vi "CreateIntegerArray.vi"(11 "Inputs":T1 {"Spacing" items=["Linear", "Logarithmic"]}) -> (3 "Output Array":dbl[](array[numeric]))   [LabVIEW 2014]
uses:
  <vilib>/imath/engines/lvmath2/RunTimeEngine/Managers/WorkSpace/UID Generator.vi
  <vilib>/imath/engines/lvmath2/RunTimeEngine/RunTimeType/NIMS_RunTimeType_From StrictType (excl LVString).vi
  <instcachedir>/0/NIMS_RunTimeType_From StrictType (excl LVString)_15A5391EEA9C4AACB9955AC755B83D29.lvgen/NIMS_RunTimeType_From StrictType (excl LVString)_15A5391EEA9C4AACB9955AC755B83D29_000.vi
  <vilib>/imath/engines/lvmath2/RunTimeEngine/LocalVariableDefStatement/MC_LocalVariableDefStatement_Display.vi
  <vilib>/imath/engines/lvmath2/RunTimeEngine/RangeToken/NIMS_Range.vi
  <instcachedir>/0/NIMS_Range_9BCE657718DF4976A877346C61F22738.lvgen/NIMS_Range_9BCE657718DF4976A877346C61F22738_000.vi
  <vilib>/imathl/engines/lvmath/Functions/Error Handling/Create Error.vi
  <vilib>/imath/engines/lvmath2/RunTimeEngine/Managers/SymbolTable/Clear UID.vi
  <vilib>/imath/engines/lvmath2/RunTimeEngine/NodeEndStatement/NIMS_NodeEndStatement_Output.vi
  <instcachedir>/0/NIMS_NodeEndStatement_Output_53EC0D466D134D7ABD903AC30B43404B.lvgen/NIMS_NodeEndStatement_Output_53EC0D466D134D7ABD903AC30B43404B_005.vi
  <vilib>/imath/engines/lvmath2/RunTimeEngine/ErrorHandling/NIMS_Finalize Error.vi
  <vilib>/imath/engines/lvmath2/RunTimeEngine/Managers/SymbolTable/NIMS_WorkSpace.lvlib
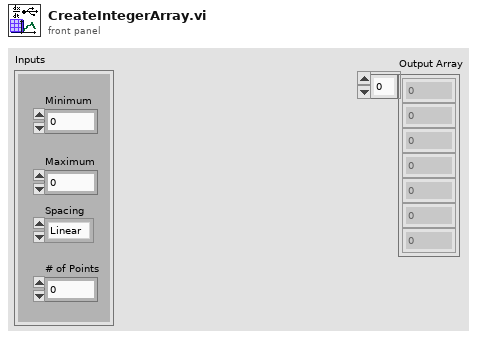
[diagram p1: front panel]
types:
  T1 = cluster{"Minimum":dbl, "Maximum":dbl, "# of Points":dbl, "Spacing":u16}
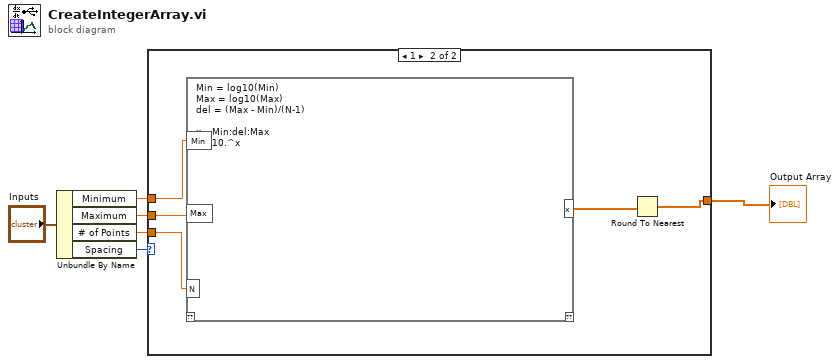
[diagram p0: block diagram]
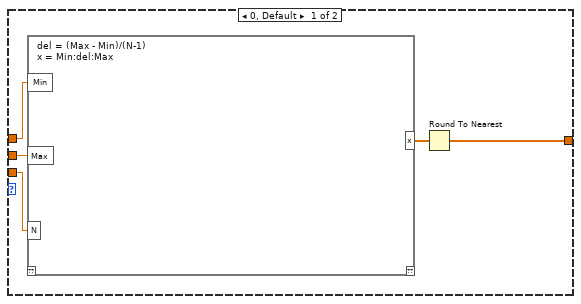
[diagram p2: hidden frame]
diagram:
  n1 = Unbundle By Name("Inputs") -> ("Minimum"=w1:dbl, "Maximum"=w2:dbl, "# of Points"=w3:dbl, "Spacing"=w4:u16)
  n2 = case shown="1" w4 {
    tunnel: [w10 w82] -> w6
    tunnel: w3 -> [w9 w84]
    tunnel: w2 -> [w8 w85]
    tunnel: w1 -> [w7 w86]
    frame 0, Default {
      n3 = mathscript code="del = (Max - Min)/(N-1)\nx = Min:del:Max"("Min"=w7, "Max"=w8, "N"=w9) -> ("x"=w11:dbl[])  [unwired: 1 in, 1 out]
      n4 = Round To Nearest(number=w11) -> (nearest integer value=w10:dbl[])
    }
    frame 1 {
      n5 = mathscript code="Min = log10(Min)\nMax = log10(Max)\ndel = (Max - Min)/(N-1)\n\nx= Min:del:Max\nx= 10.^x"("Min"=w86, "Max"=w85, "N"=w84) -> ("x"=w83:dbl[])  [unwired: 1 in, 1 out]
      n6 = Round To Nearest(number=w83) -> (nearest integer value=w82:dbl[])
    }
  }
  "Output Array" <- w6
